vi "_PC_NS_Wfm_Process.vi"(7 "Wfm_Type":T1, 8 "error in (no error)":errorcluster, 10 "WfmData_U64 in":u64[](array[numeric])) -> (0 "error out":errorcluster)   [LabVIEW 2018]
uses:
  Daemon/RecipeEditor/Ctl/WfmCmd_Type.ctl
  RT/PublicSubVI/Ctl/_ctl_RT_NS_Status.ctl
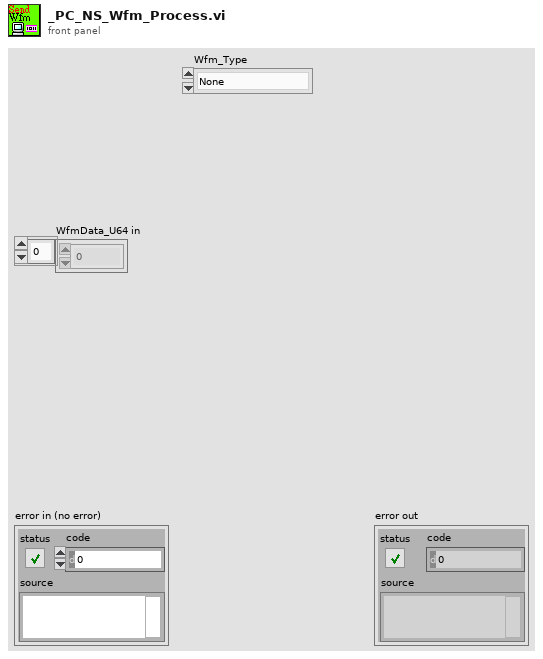
[diagram p1: front panel]
types:
  T1 = typedef "WfmCmd_Type.ctl" = enum8{"None", "WFM", "EventCodes"}
  T2 = typedef "_ctl_RT_NS_Status.ctl" = enum8{"Idle", "Init", "Connected", "Stop"}
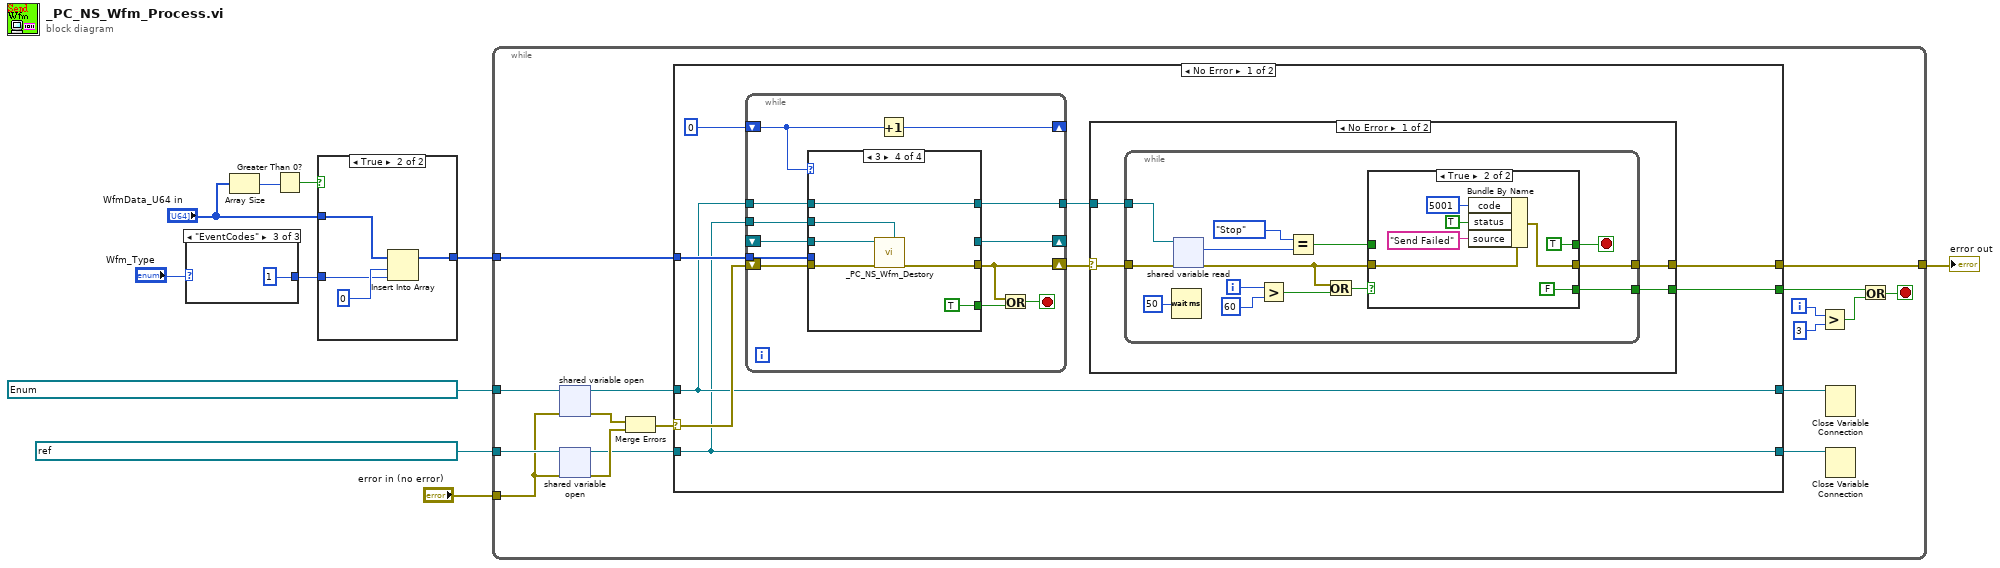
[diagram p0: block diagram]
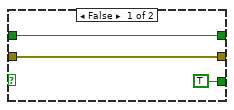
[diagram p2: hidden frame]
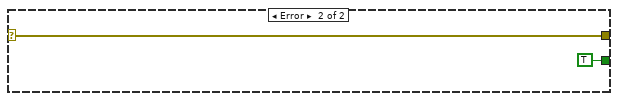
[diagram p3: hidden frame]
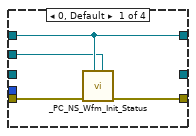
[diagram p4: hidden frame]
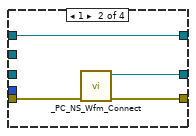
[diagram p5: hidden frame]
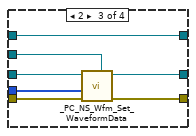
[diagram p6: hidden frame]
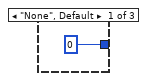
[diagram p8: hidden frame]
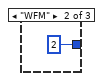
[diagram p9: hidden frame]
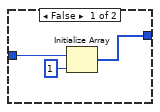
[diagram p10: hidden frame]
diagram:
  w9 = refnum<k21> "ni.var.psp://NI-sbRIO/_RT_CtrlLoop_WfmData_Variable/Wfm_Connect_Status" items=["Idle", "Init", "Connected", "Stop"] ("shared variable refnum in")
  n1 = case shown="\"EventCodes\"" "Wfm_Type" {
    tunnel: [u64 0 u64 2 u64 1] -> w6
    frame "None", Default {
    }
    frame "WFM" {
    }
    frame "EventCodes" {
    }
  }
  n2 = Array Size(array="WfmData_U64 in") -> (size(s)=w2:i32)
  n3 = Greater Than 0?(x=w2) -> (x > 0?=w3:bool)
  n4 = case shown="True" w3 {
    tunnel: "WfmData_U64 in" -> [_ w20]
    tunnel: w6 -> [w16 w18]
    tunnel: [w14 w17] -> w1
    frame False {
      n5 = Initialize Array(w16, 1 ("dimension size")) -> (w14:u64[])
    }
    frame True {
      n6 = Insert Into Array(array=w20, index=0, new element=w18) -> (w17:u64[])
    }
  }
  n7 = while {
    tunnel: refnum<k21> "ni.var.psp://NI-sbRIO/_RT_CtrlLoop_WfmData_Variable/Wfm_Stop_Bool" ("shared variable refnum in") -> [w37]
    tunnel: w9 -> [w36]
    tunnel: "error in (no error)" -> [w28]
    tunnel: [w27] -> w7
    tunnel: w1 -> [w22]
    i -> [w24]
    stop <- w21 stop-if-true
    n8 = shared-variable-open(w36, w28) -> (w31:refnum<k21>, w35:errorcluster)
    n9 = shared-variable-open(w37, w28) -> (w32:refnum<k21>, w34:errorcluster)
    n10 = Merge Errors(w35, w34) -> (w33:errorcluster)
    n11 = case shown="No Error" w33 {
      selector: w33 -> [w41 w112]
      tunnel: w32 -> [w39 w110]
      tunnel: w31 -> [w40 w111]
      tunnel: [w39 w110] -> w30
      tunnel: [w40 w111] -> w29
      tunnel: [w42 w112] -> w27
      tunnel: [w43 _] -> w23
      tunnel: w22 -> [w45 _]
      frame No Error {
        n12 = while {
          shift-right: [w87] -> _
          shift-left: 0 -> [w86]
          shift-right: [w85] -> _
          shift-left: _ -> [w84]
          tunnel: w45 -> [w83]
          shift-right: [w81] -> w44
          shift-left: w41 -> [w88]
          tunnel: w40 -> [w79]
          tunnel: w39 -> [w78]
          tunnel: [w77] -> w38
          stop <- w80 stop-if-true
          n13 = case shown="3" w86 {
            tunnel: w88 -> [w92 w96 w103 w108]
            tunnel: [w91 w95 w102 w107] -> w81
            tunnel: [_ w94 w101 _] -> w85
            tunnel: w84 -> [_ _ w100 w109]
            tunnel: w83 -> [_ _ w99 _]
            tunnel: [_ _ _ TRUE] -> w82
            tunnel: w79 -> [w90 w93 w98 w105]
            tunnel: w78 -> [w89 _ w97 w104]
            tunnel: [w90 w93 w98 w105] -> w77
            frame 0, Default {
              n14 = call "_PC_NS_Wfm_Init_Status.vi"("wfm stop bool"=w89, "wfm connect status"=w90, "error IO"=w92) -> ("error Out"=w91:errorcluster)  [unwired: 8 in]
            }
            frame 1 {
              n15 = call "_PC_NS_Wfm_Connect.vi"("error In"=w96) -> ("error Out"=w95:errorcluster, "writer name Out"=w94:refnum<k21>)  [unwired: 9 in]
            }
            frame 2 {
              n16 = call "_PC_NS_Wfm_Set_WaveformData.vi"("wfm stop bool"=w97, "error In"=w103, "WfmData_U64 in"=w99, "writer name In"=w100) -> ("error Out"=w102:errorcluster, "writer name Out"=w101:refnum<k21>)  [unwired: 6 in]
            }
            frame 3 {
              n17 = call "_PC_NS_Wfm_Destory.vi"("wfm stop bool"=w104, "error in (no error)"=w108, "writer name In"=w109) -> ("error out"=w107:errorcluster)  [unwired: 8 in]
            }
          }
          n18 = Increment(x=w86) -> (x+1=w87:i32)
          n19 = Or(x=w81, y=w82) -> (x .or. y?=w80:bool)
        }
        n20 = case shown="No Error" w44 {
          selector: w44 -> [w50 w76]
          tunnel: [w49 w76] -> w42
          tunnel: [w48 TRUE] -> w43
          tunnel: w38 -> [w47 _]
          frame No Error {
            n21 = while {
              tunnel: w50 -> [w53]
              tunnel: [w59] -> w49
              tunnel: [w55] -> w48
              tunnel: w47 -> [w54]
              i -> [w62]
              stop <- w57 stop-if-true
              n22 = Wait (ms)(milliseconds to wait=u32 50) -> ()  [unwired: 1 out]
              n23 = shared-variable-read(w54, w53) -> (w51:errorcluster, w52:T2)  [unwired: 2 out]
              n24 = Greater?(x=w62, y=60) -> (0:w60:bool)
              n25 = Equal?(x=_ctl_RT_NS_Status."Stop", y=w52) -> (x = y?=w56:bool)
              n26 = Or(x=w51, y=w60) -> (x .or. y?=w58:bool)
              n27 = case shown="True" w58 {
                tunnel: [w66 w73] -> w59
                tunnel: w51 -> [w66 w74]
                tunnel: [w67 TRUE] -> w57
                tunnel: w56 -> [w67 _]
                tunnel: [TRUE FALSE] -> w55
                frame False {
                }
                frame True {
                  n28 = Bundle By Name(cluster=w74, "code"=5001, "status"=TRUE, "source"="Send Failed") -> (w73:errorcluster)
                }
              }
            }
          }
          frame Error {
          }
        }
      }
      frame Error {
      }
    }
    n29 = Greater?(x=w24, y=3) -> (0:w25:bool)
    n30 = Close Variable Connection(11:w29) -> ()  [unwired: 1 in, 1 out]
    n31 = Close Variable Connection(11:w30) -> ()  [unwired: 1 in, 1 out]
    n32 = Or(x=w23, y=w25) -> (x .or. y?=w21:bool)
  }
  "error out" <- w7
